vi "General_Setup_string.vi"() -> (0 "Output string":string)   [LabVIEW 2020]
uses:
  Controls/Graph_Type.ctl
  Controls/Tunnel_Coordinates.ctl
  Globals/Preference_global.vi
  Globals/Meas_global.vi
  Globals/Extra_Commands_Global.vi
  Globals/Trav_pos_global.vi
panel:
  in  "Plot Type":T1=enum."Voltage trace"
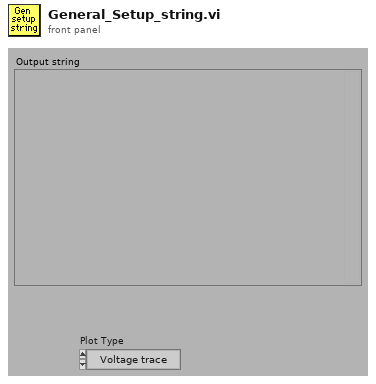
[diagram p1: front panel]
types:
  T1 = typedef "Graph_Type.ctl" = enum16{"Show no graph", "Voltage trace", "Velocity trace", "Vel histogram", "Spectrum", "f.E(f) v Log f", "Auto-Corr"}
  T2 = typedef "Tunnel_Coordinates.ctl" = enum16{"Work in Tunnel Coordinates", "Work in Model Coordinates"}
  T3 = enum16{"From String to Cluster", "From Cluster to String"}
  T4 = cluster{"Plot 1":u16, "Plot 2":u16, "Save graph":u16, "Plot Type":T1}
  T5 = enum16{"Save no data", "Save data in new files", "Save data in existing files"}
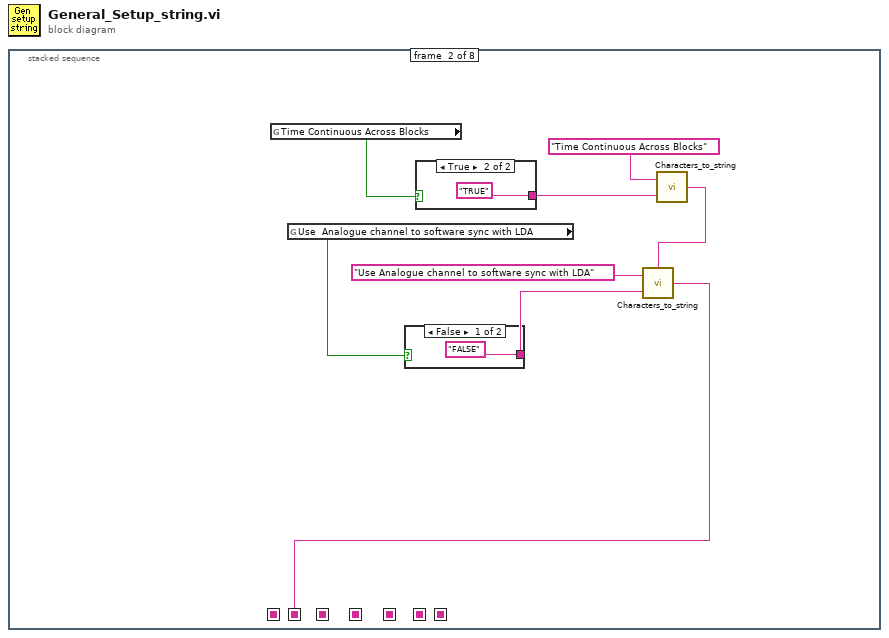
[diagram p0: block diagram]
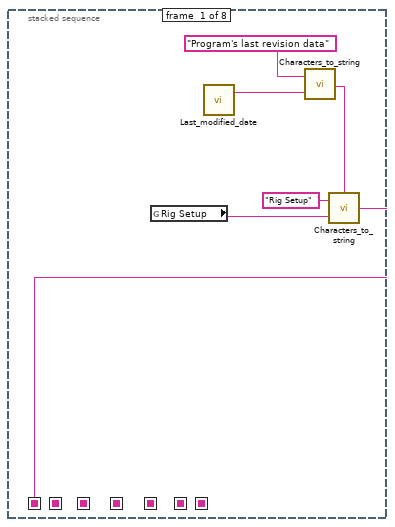
[diagram p2: hidden frame]
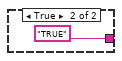
[diagram p3: hidden frame]
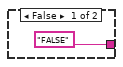
[diagram p4: hidden frame]
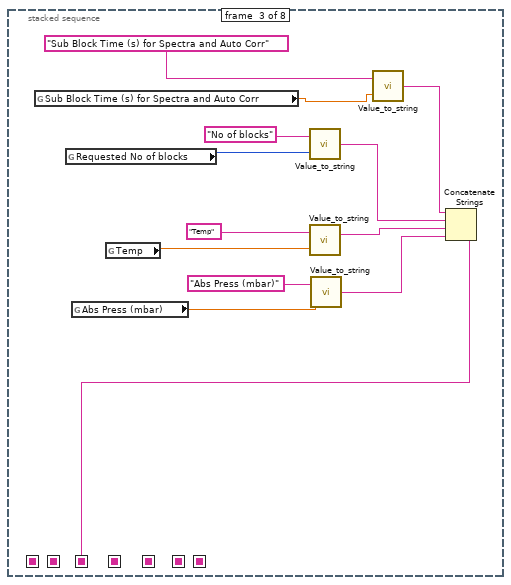
[diagram p5: hidden frame]
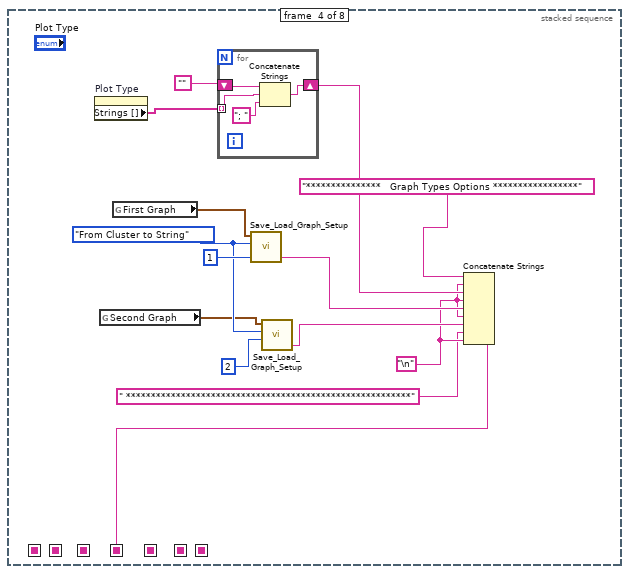
[diagram p6: hidden frame]
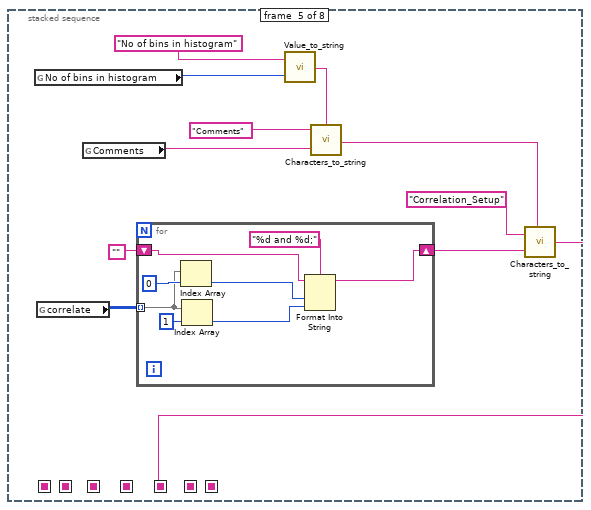
[diagram p7: hidden frame]
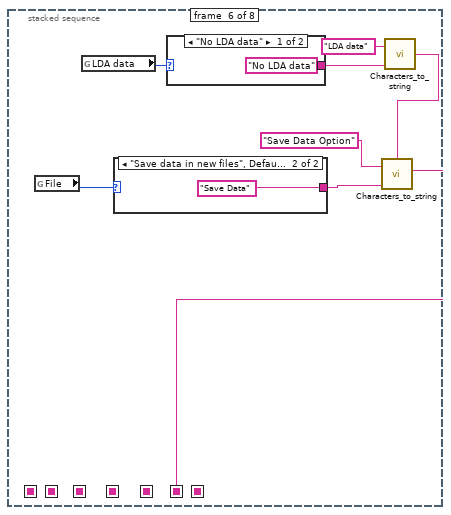
[diagram p8: hidden frame]
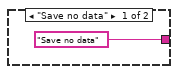
[diagram p9: hidden frame]
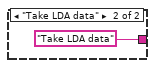
[diagram p10: hidden frame]
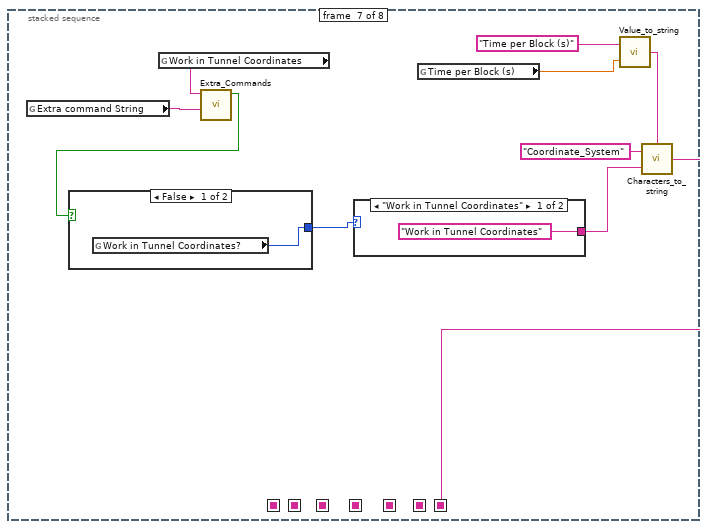
[diagram p11: hidden frame]
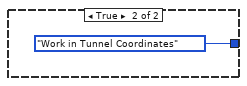
[diagram p12: hidden frame]
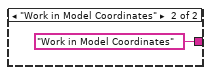
[diagram p13: hidden frame]
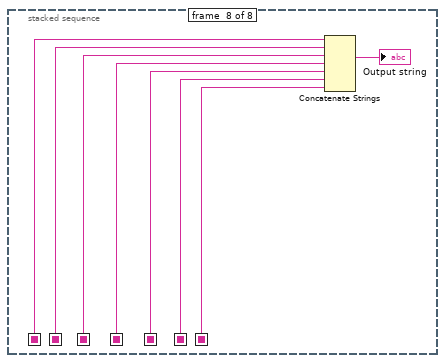
[diagram p14: hidden frame]
diagram:
  n1 = stacked-sequence {
    seq-local: [_ _ w29 _ _ _ _ _] -> [_ _ _ _ _ _ _ w102]
    seq-local: [_ w7 _ _ _ _ _ _] -> [_ _ _ _ _ _ _ w101]
    seq-local: [_ _ _ _ _ w69 _ _] -> [_ _ _ _ _ _ _ w97]
    seq-local: [_ _ _ _ _ _ w81 _] -> [_ _ _ _ _ _ _ w96]
    seq-local: [_ _ _ w45 _ _ _ _] -> [_ _ _ _ _ _ _ w99]
    seq-local: [_ _ _ _ w50 _ _ _] -> [_ _ _ _ _ _ _ w98]
    seq-local: [w1 _ _ _ _ _ _ _] -> [_ _ _ _ _ _ _ w95]
    frame #0 {
      n2 = global read "Preference_global.vi" "Rig Setup"() -> (w5:string)
      n3 = call "Last_modified_date.vi"() -> ("concatenatedRevisions"=w3:string)  [unwired: 1 in, 1 out]
      n4 = call "Characters_to_string.vi"("Characters to write"=w3, "Label for characters"="Program's last revision data") -> ("Output string"=w2:string)  [unwired: 1 in]
      n5 = call "Characters_to_string.vi"("stringIn"=w2, "Characters to write"=w5, "Label for characters"="Rig Setup") -> ("Output string"=w1:string)
    }
    frame #1 {
      n6 = global read "Meas_global.vi" "Time Continuous Across Blocks"() -> (w12:bool)
      n7 = global read "Meas_global.vi" "Use  Analogue channel to software sync with LDA"() -> (w10:bool)
      n8 = case shown="False" w10 {
        tunnel: ["FALSE" "TRUE"] -> w9
        frame False {
        }
        frame True {
        }
      }
      n9 = case shown="True" w12 {
        tunnel: ["FALSE" "TRUE"] -> w11
        frame False {
        }
        frame True {
        }
      }
      n10 = call "Characters_to_string.vi"("Characters to write"=w11, "Label for characters"="Time Continuous Across Blocks") -> ("Output string"=w8:string)  [unwired: 1 in]
      n11 = call "Characters_to_string.vi"("stringIn"=w8, "Characters to write"=w9, "Label for characters"="Use Analogue channel to software sync with LDA") -> ("Output string"=w7:string)
    }
    frame #2 {
      n12 = global read "Meas_global.vi" "Sub Block Time (s) for Spectra and Auto Corr"() -> (w19:dbl)
      n13 = global read "Meas_global.vi" "Requested No of blocks"() -> (w30:i32)
      n14 = global read "Meas_global.vi" "Abs Press (mbar)"() -> (w26:dbl)
      n15 = global read "Meas_global.vi" "Temp"() -> (w25:dbl)
      n16 = call "Value_to_string.vi"("Value"=w30, "Label for value"="No of blocks") -> ("Output string"=w22:string)  [unwired: 1 in]
      n17 = call "Value_to_string.vi"("Value"=w25, "Label for value"="Temp") -> ("Output string"=w24:string)  [unwired: 1 in]
      n18 = call "Value_to_string.vi"("Value"=w26, "Label for value"="Abs Press (mbar)") -> ("Output string"=w23:string)  [unwired: 1 in]
      n19 = call "Value_to_string.vi"("Value"=w19, "Label for value"="Sub Block Time (s) for Spectra and Auto Corr") -> ("Output string"=w20:string)  [unwired: 1 in]
      n20 = Concatenate Strings(w20, w22, w24, w23) -> (w29:string)
    }
    frame #3 {
      w35 = "\n"
      w42 = T3."From Cluster to String" ("Mode")
      n21 = property on="Plot Type" class="Enum (strict)"() -> ("Strings []"=w37:string[])  [unwired: 2 in, 2 out]
      n22 = global read "Meas_global.vi" "Second Graph"() -> (w41:T4)
      n23 = global read "Meas_global.vi" "First Graph"() -> (w38:T4)
      n24 = for {
        shift-right: [w48] -> w36
        shift-left: "" -> [w49]
        tunnel: w37 -> [w47] mode=indexing
        n25 = Concatenate Strings(w49, w47, "; " ("string")) -> (w48:string)
      }
      n26 = call "Save_Load_Graph_Setup.vi"("Graph Number"=1, "Mode"=w42, "Graph in"=w38) -> ("Setup String Out"=w39:string)  [unwired: 1 in, 2 out]
      n27 = call "Save_Load_Graph_Setup.vi"("Graph Number"=2, "Mode"=w42, "Graph in"=w41) -> ("Setup String Out"=w40:string)  [unwired: 1 in, 2 out]
      n28 = Concatenate Strings("***************   Graph Types Options *****************", w35, w36, w35, w39, w35, w40, " *********************************************************" ("string"), w35) -> (w45:string)
    }
    frame #4 {
      n29 = global read "Meas_global.vi" "No of bins in histogram"() -> (w59:i32)
      n30 = global read "Meas_global.vi" "correlate"() -> (w56:i32[][])
      n31 = global read "Meas_global.vi" "Comments"() -> (w57:string)
      n32 = for {
        tunnel: w56 -> [w66] mode=indexing
        shift-right: [w62] -> w53
        shift-left: "" -> [w63]
        n33 = Index Array(array=w66, index=0) -> (element=w65:i32)
        n34 = Index Array(array=w66, index=1) -> (element=w64:i32)
        n35 = Format Into String(format string="%d and %d;", initial string=w63, w65, w64) -> (resulting string=w62:string)  [unwired: 1 in, 1 out]
      }
      n36 = call "Value_to_string.vi"("Value"=w59, "Label for value"="No of bins in histogram") -> ("Output string"=w52:string)  [unwired: 1 in]
      n37 = call "Characters_to_string.vi"("stringIn"=w52, "Characters to write"=w57, "Label for characters"="Comments") -> ("Output string"=w51:string)
      n38 = call "Characters_to_string.vi"("stringIn"=w51, "Characters to write"=w53, "Label for characters"="Correlation_Setup") -> ("Output string"=w50:string)
    }
    frame #5 {
      n39 = global read "Meas_global.vi" "File"() -> (w73:T5)
      n40 = global read "Meas_global.vi" "LDA data"() -> (w74:enum16{"No LDA data", "Take LDA data"})
      n41 = case shown="\"Save data in new files\", Default" w73 {
        tunnel: ["Save no data" "Save Data"] -> w71
        frame "Save no data" {
        }
        frame "Save data in new files", Default {
        }
      }
      n42 = case shown="\"No LDA data\"" w74 {
        tunnel: ["No LDA data" "Take LDA data"] -> w75
        frame "No LDA data" {
        }
        frame "Take LDA data" {
        }
      }
      n43 = call "Characters_to_string.vi"("Characters to write"=w75, "Label for characters"="LDA data") -> ("Output string"=w70:string)  [unwired: 1 in]
      n44 = call "Characters_to_string.vi"("stringIn"=w70, "Characters to write"=w71, "Label for characters"="Save Data Option") -> ("Output string"=w69:string)
    }
    frame #6 {
      n45 = global read "Meas_global.vi" "Extra command String"() -> (w85:string)
      n46 = global read "Extra_Commands_Global.vi" "Work in Tunnel Coordinates"() -> (w86:string)
      n47 = call "Extra_Commands.vi"("String to Search"=w85, "Command"=w86) -> ("Command Found"=w84:bool)  [unwired: 1 in, 4 out]
      n48 = case shown="False" w84 {
        tunnel: [w91 Tunnel_Coordinates."Work in Tunnel Coordinates" ("Work in Tunnel Coordinates?")] -> w83
        frame False {
          n49 = global read "Trav_pos_global.vi" "Work in Tunnel Coordinates?"() -> (w91:T2)
        }
        frame True {
        }
      }
      n50 = case shown="\"Work in Tunnel Coordinates\"" w83 {
        tunnel: ["Work in Tunnel Coordinates" "Work in Model Coordinates"] -> w90
        frame "Work in Tunnel Coordinates" {
        }
        frame "Work in Model Coordinates" {
        }
      }
      n51 = global read "Meas_global.vi" "Time per Block (s)"() -> (w87:dbl)
      n52 = call "Value_to_string.vi"("Value"=w87, "Label for value"="Time per Block (s)") -> ("Output string"=w82:string)  [unwired: 1 in]
      n53 = call "Characters_to_string.vi"("stringIn"=w82, "Characters to write"=w90, "Label for characters"="Coordinate_System") -> ("Output string"=w81:string)
    }
    frame #7 {
      n54 = Concatenate Strings(w95, w101, w102, w99, w98, w97, w96) -> (→"Output string":string)
    }
  }
